vi "EditOptions.vi"(8 "error in":errorcluster, 11 "SequenceNode in":refnum<class "MainCategoryNode.lvclass">) -> (0 "error out":errorcluster, 1 "edit options":T1, 2 "subnodes class":T2, 3 "SequenceNode out":refnum<class "MainCategoryNode.lvclass">)   [LabVIEW 2015, in "MainCategoryNode.lvclass"]
doc: "This VI Contains the options for the Menu that will be displayed when doing right click on an item\nThe subnodes class configures which nodes can be added to this nodes\nAnd the edit options determine which options are available for the node.\n\nThis configuration is stored in this VI in case some dynamic configuration is required for the menu options or subnodes.\n\nAll VIs must overide this methodCopyright 2017 National Instruments Corporation\n\nLicensed under the Apache License, Version 2.0 (the \"License\"); you may not use this file except in compliance with the License. You may obtain a copy of the License at http://www.apache.org/licenses/LICENSE-2.0\nUnless required by applicable law or agreed to in writing, software distributed under the License is distributed on an \"AS IS\" BASIS, WITHOUT WARRANTIES OR CONDITIONS OF ANY KIND, either express or implied. See the License for the specific language governing permissions and limitations under the License."
uses:
  MainCategoryNode.lvclass
  <vilib>/NI/Configuration Framework/Node/SubNodeCluster.ctl
  <vilib>/NI/Configuration Framework/Node/NodeMenuOptions.ctl
  <vilib>/NI/Configuration Framework/Node/NISE_CEF_Node.lvclass
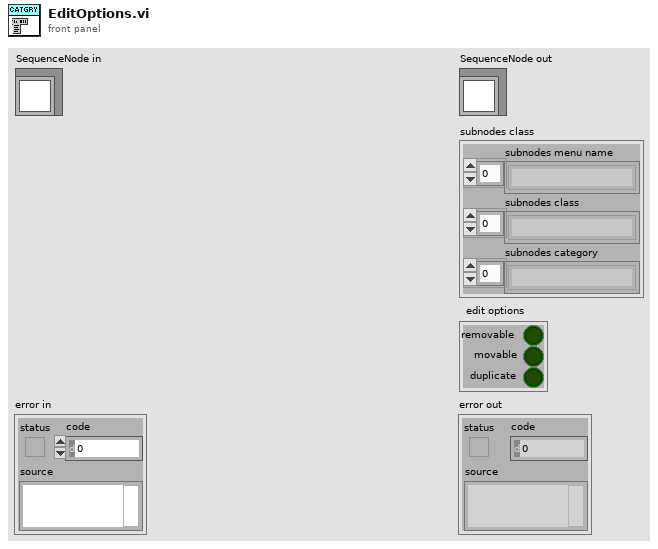
[diagram p1: front panel]
types:
  T1 = typedef "NISE_CEF_Node.lvclass/NodeMenuOptions.ctl" = cluster{"removable":bool, "movable":bool, "duplicate":bool}
  T2 = typedef "NISE_CEF_Node.lvclass/SubNodeCluster.ctl" = cluster{"subnodes menu name":string[], "subnodes class":string[], "subnodes category":string[]}
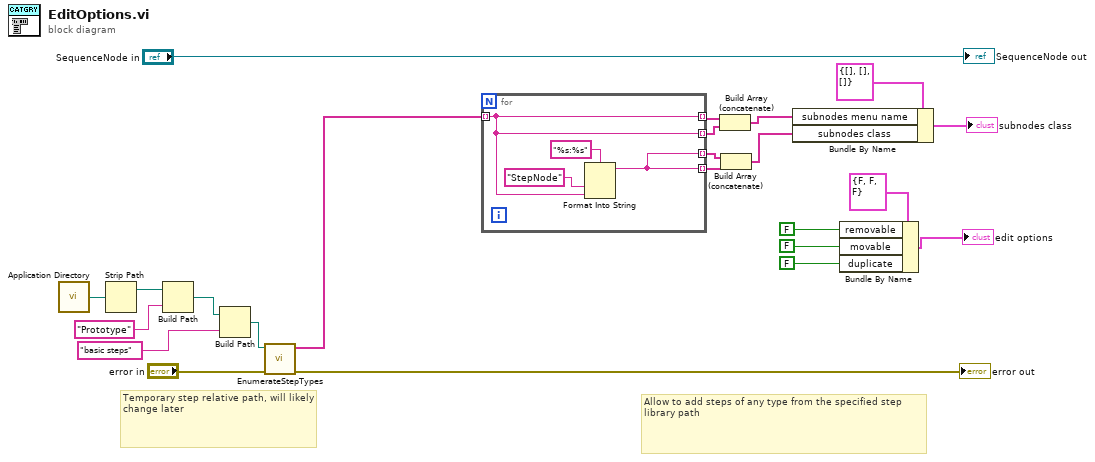
[diagram p0: block diagram]
diagram:
  # "Temporary step relative path, will likely change later"
  # "Allow to add steps of any type from the specified step library path"
  n1 = call <vilib>:"Application Directory.vi"() -> ("Application Directory"=w14:path)
  n2 = Strip Path(path=w14) -> (stripped path=w13:path)  [unwired: 1 out]
  n3 = Build Path(base path=w13, name or relative path="Prototype") -> (appended path=w11:path)
  n4 = Build Path(base path=w11, name or relative path="basic steps") -> (appended path=w8:path)
  n5 = call "EnumerateStepTypes.vi"("error in (no error)"="error in", "Step Classes Folder"=w8) -> ("error out"=→"error out":errorcluster, "Step Names"=w7:string[])  [unwired: 8 in]
  n6 = for {
    tunnel: w7 -> [w24] mode=indexing
    tunnel: [w27] -> w3 mode=indexing
    tunnel: [w27] -> w2 mode=indexing
    tunnel: [w24] -> w6 mode=indexing
    tunnel: [w24] -> w5 mode=indexing
    n7 = Format Into String(format string="%s:%s", "StepNode", w24) -> (resulting string=w27:string)  [unwired: 2 in, 1 out]
  }
  n8 = Build Array (concatenate)(w6, w5) -> (w4:string[])
  n9 = Build Array (concatenate)(w2, w3) -> (w1:string[])
  n10 = Bundle By Name(cluster=T2 {"subnodes menu name"=[], "subnodes class"=[], "subnodes category"=[]} ("subnodes class"), "subnodes menu name"=w4, "subnodes class"=w1) -> (→"subnodes class":T2)
  n11 = Bundle By Name(cluster=T1 {"removable"=FALSE, "movable"=FALSE, "duplicate"=FALSE} ("edit options"), "removable"=FALSE ("Removable"), "movable"=FALSE ("Movable"), "duplicate"=FALSE ("Duplicate")) -> (→"edit options":T1)
  "SequenceNode out" <- "SequenceNode in"
